vi "Start IP Reporter.vi"(4 "ignore Gateway IP?(T)":bool=TRUE, 6 "Load From File(F)":bool, 8 "error in (no error)":errorcluster, 10 "Init Information":string, 11 "Setttings":T1={"address"="234.5.6.7", "receiver port"=58432, "Ignore Gateway IP"=TRUE, "HostName"=""}) -> (0 "error out":errorcluster, 3 "Information Notifier":refnum<notifier>)   [LabVIEW 2017]
uses:
  _Typedef/Def-IniSettings -- Cluster.ctl
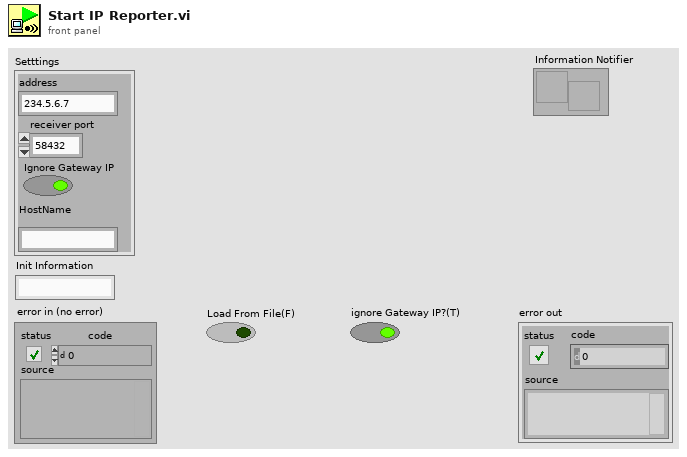
[diagram p1: front panel]
types:
  T1 = typedef "Def-IniSettings -- Cluster.ctl" = cluster{"address":string, "receiver port":u16, "Ignore Gateway IP":bool, "HostName":string}
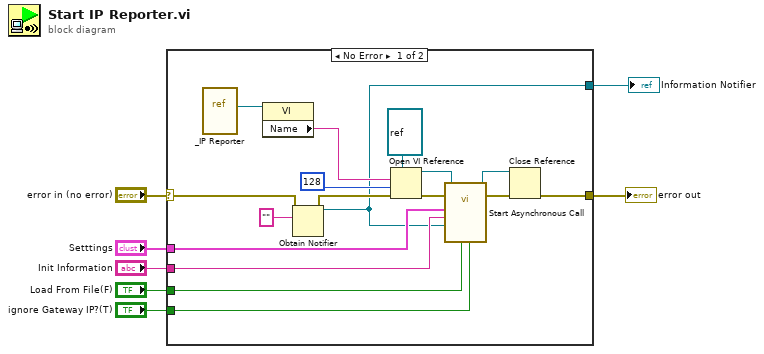
[diagram p0: block diagram]
diagram:
  n1 = case shown="No Error" "error in (no error)" {
    selector: "error in (no error)" -> [w24 w25]
    tunnel: [w17 w25] -> w6
    tunnel: "Setttings" -> [w12 _]
    tunnel: "Load From File(F)" -> [w11 _]
    tunnel: "ignore Gateway IP?(T)" -> [w10 _]
    tunnel: "Init Information" -> [w9 _]
    tunnel: [w8 _] -> w1
    frame No Error {
      n2 = vi-ref "_IP Reporter.vi"() -> (w22:refnum<vi>)
      n3 = property class="VI"(reference=w22) -> ("Name"=w21:string)  [unwired: 1 in, 2 out]
      n4 = Obtain Notifier(notification data type="", error in (no error)=w24) -> (notifier out=w8:refnum<notifier>, error out=w14:errorcluster)  [unwired: 2 in, 1 out]
      n5 = Open VI Reference(type specifier VI Refnum (for type only)=refnum<vi> refnum, vi path=w21, options=128, error in (no error)=w14) -> (vi reference=w15:refnum<vi>, error out=w23:errorcluster)  [unwired: 2 in]
      n6 = call-by-ref "Start Asynchronous Call"(reference=w15, error in=w23, "ignore Gateway IP?(T)"=w10, "Load From File(F)"=w11, "notifier"=w8, "Init-Information"=w9, "Setttings"=w12) -> (reference out=w16:refnum<vi>, error out=w19:errorcluster)  [unwired: 6 in, 1 out]
      n7 = Close Reference(reference=w16, error in (no error)=w19) -> (error out=w17:errorcluster)
    }
    frame Error {
    }
  }
  "error out" <- w6
  "Information Notifier" <- w1
